vi "检测CTR.vi"(0 "Data In":T3=enum."Runing" caption="数据输入", 2 "Display State In":T2={"Data"=enum."Runing"} caption="显示状态输入", 3 "Container State":T4 caption="容器状态") -> (6 "Data Out":T3=enum."Runing" caption="数据输出", 7 "Display State Out":T2={"Data"=enum."Runing"} caption="显示状态输出", 8 "Action":T1 caption="动作")   [LabVIEW 2020, in "检测CTR.xctl"]
uses:
  <vilib>/_xctls/Container State.ctl
  <vilib>/_xctls/Action.ctl
  <vilib>/_xctls/XControlSupport.lvlib
panel:
  out "字符串 2":string
  out "字符串":string
  out "颜色盒":u32(colorbox)
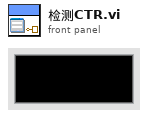
[diagram p1: front panel]
types:
  T1 = typedef "XControlSupport.lvlib/Action.ctl" = cluster{"Data Changed?":bool, "State Changed?":bool, "Action Name":string}
  T2 = typedef "检测CTR.xctl/检测CTR状态.ctl" = cluster{"Data":T3}
  T3 = typedef "检测CTR.xctl/检测CTR数据.ctl" = enum16{"Idle", "Runing", "Pass", "Faild", "Skip"}
  T4 = typedef "XControlSupport.lvlib/Container State.ctl" = cluster{"Indicator?":bool, "Run Mode?":bool, " Refnum":refnum<vi>}
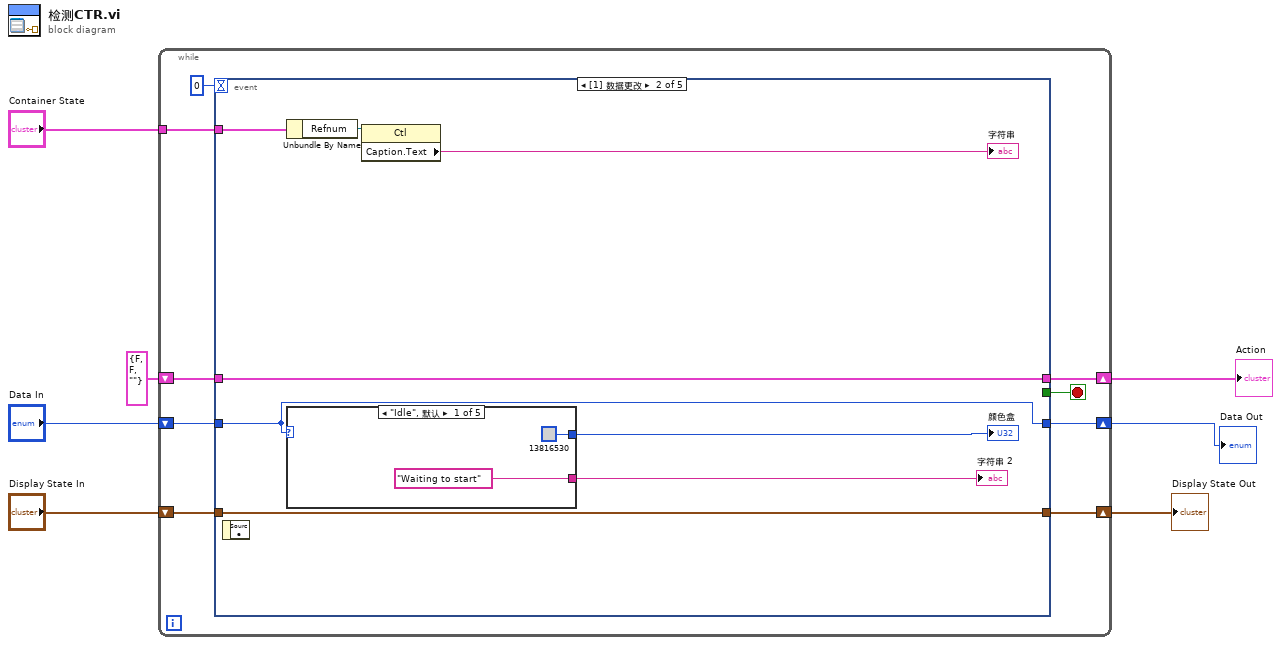
[diagram p0: block diagram]
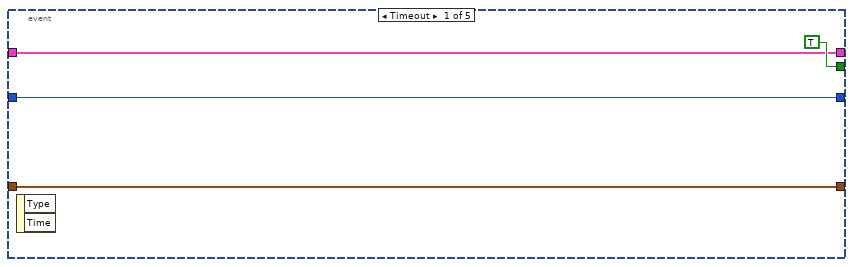
[diagram p2: hidden frame]
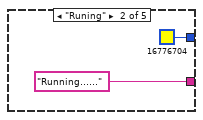
[diagram p3: hidden frame]
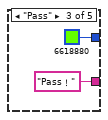
[diagram p4: hidden frame]
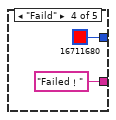
[diagram p5: hidden frame]
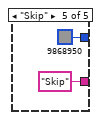
[diagram p6: hidden frame]
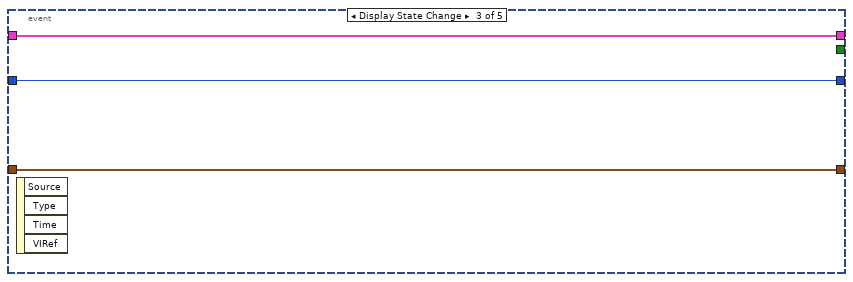
[diagram p7: hidden frame]
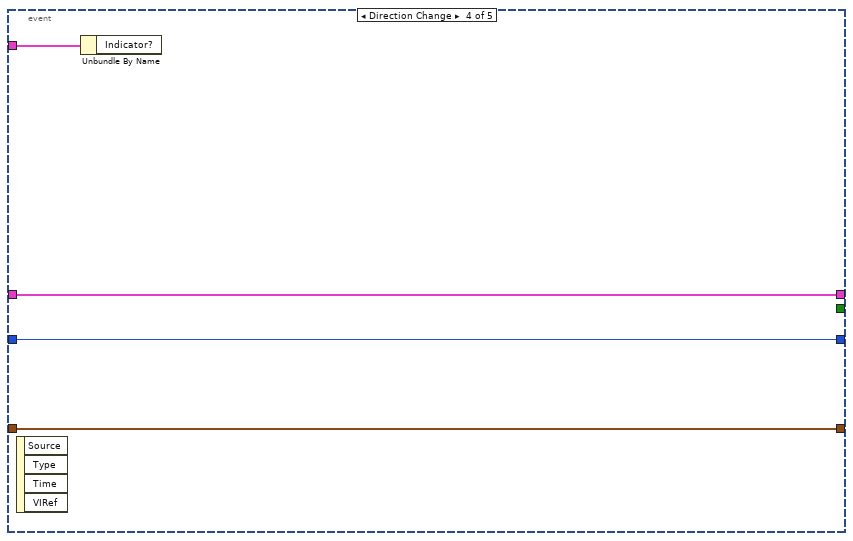
[diagram p8: hidden frame]
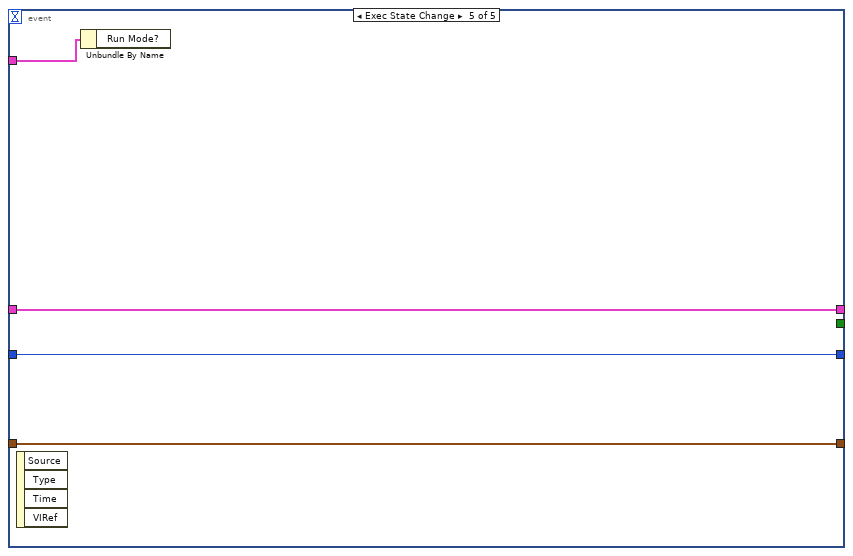
[diagram p9: hidden frame]
diagram:
  n1 = while {
    shift-right: [w15] -> w4
    shift-left: "Display State In" -> [w16]
    tunnel: "Container State" -> [w12]
    shift-right: [w10] -> w7
    shift-left: "Data In" -> [w11]
    shift-right: [w8] -> w2
    shift-left: T1 {"Data Changed?"=FALSE, "State Changed?"=FALSE, "Action Name"=""} ("Action") -> [w9]
    stop <- w14 stop-if-true
    n2 = event shown="[1] 数据更改" {
      selector: _ -> [_ _ _ _ _]
      dyn-events: _ -> [_ _ _ _ _]
      timeout: 0 -> [_ _ _ _ _]
      tunnel: w16 -> [w18 w28 w41 w44 w48]
      tunnel: [w18 w28 w41 w44 w48] -> w15
      tunnel: [TRUE _ _ _ _] -> w14
      tunnel: w12 -> [_ w24 _ w45 w49]
      tunnel: w11 -> [w17 w26 w40 w43 w47]
      tunnel: [w17 w26 w40 w43 w47] -> w10
      tunnel: [w19 w27 w39 w42 w46] -> w8
      tunnel: w9 -> [w19 w27 w39 w42 w46]
      event Timeout {
        n3 = event-data() -> ()  [unwired: 1 in, 2 out]
      }
      event Data Change {
        n4 = event-data() -> ()  [unwired: 1 in, 1 out]
        n5 = Unbundle By Name(w24) -> ("Refnum"=w23:refnum<vi>)
        n6 = case shown="\"Idle\", 默认" w26 {
          tunnel: ["Waiting to start" ("字符串") "Running……" ("字符串") "Pass！" ("字符串") "Failed！" ("字符串") "Skip" ("字符串")] -> w21
          tunnel: [u32 13816530 ("颜色盒") u32 16776704 ("颜色盒") u32 6618880 ("颜色盒") u32 16711680 ("颜色盒") u32 9868950 ("颜色盒")] -> w25
          frame "Idle", Default {
          }
          frame "Runing" {
          }
          frame "Pass" {
          }
          frame "Faild" {
          }
          frame "Skip" {
          }
        }
        "颜色盒" <- w25
        "字符串 2" <- w21
        n7 = property class="Ctl"(reference=w23) -> ("Caption.Text"=→"字符串":string)  [unwired: 1 in, 2 out]
      }
      event Display State Change {
        n8 = event-data() -> ()  [unwired: 1 in, 4 out]
      }
      event Direction Change {
        n9 = event-data() -> ()  [unwired: 1 in, 4 out]
        n10 = Unbundle By Name(w45) -> ()  [unwired: 1 out]
      }
      event Exec State Change {
        n11 = event-data() -> ()  [unwired: 1 in, 4 out]
        n12 = Unbundle By Name(w49) -> ()  [unwired: 1 out]
      }
    }
  }
  "Display State Out" <- w4
  "Data Out" <- w7
  "Action" <- w2
